vi "Keithley 2002 Scan Read.vi"(1 "delay between\nbus triggers (mS)":dbl=300.0 min=0.0 step=1.0, 2 "scan operation (int:0)":u16(ring) items=["internal", "ratio", "delta"], 4 "count value":dbl=100.0 min=2.0 max=30092.0 step=1.0, 5 "delay (secs)":dbl min=0.0 max=999999.999 format="%.3f", 6 "error in":T2, 7 "timer value (secs)":dbl=0.001 min=0.001 max=999999.999 format="%.3f", 8 "source (imm:1)":u16(ring)=1 items=["hold", "immediate", "timer", "manual", "bus", "trigger link", "external"], 9 "GPIB address":string="16") -> (0 "error out":T2, 3 "measurements":T1(array[cluster]) {"measurement" format="%.6e"})   [LabVIEW 2020]
doc: "This VI is used to configure the Measure Layer (Trigger) and then read the scanning channels. The count value will control the number of measurements taken. The channels (1-10) will be scanned in order. If the count value is more than the number of channels to be scanned, the scan will repeat and read through the channels again.\n\nTo configure the scanning channels, use the Scan Config VI."
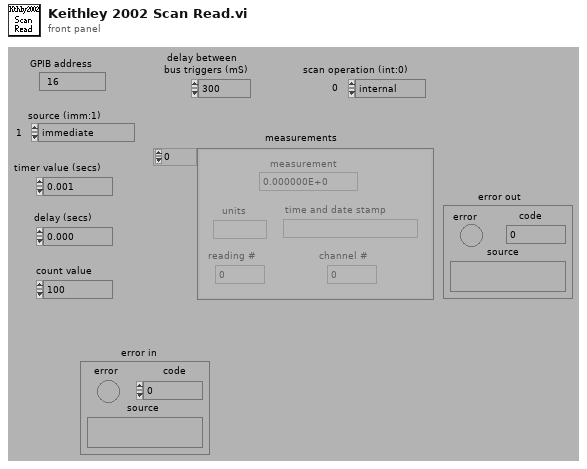
[diagram p1: front panel]
types:
  T1 = cluster{"measurement":dbl, "units":string, "time and date stamp":string, "reading #":dbl, "channel #":dbl}[]
  T2 = cluster{"error":bool, "code":i32, "source":string}
  T3 = cluster{dbl, "read buffer":string, "read buffer":string, dbl, dbl}
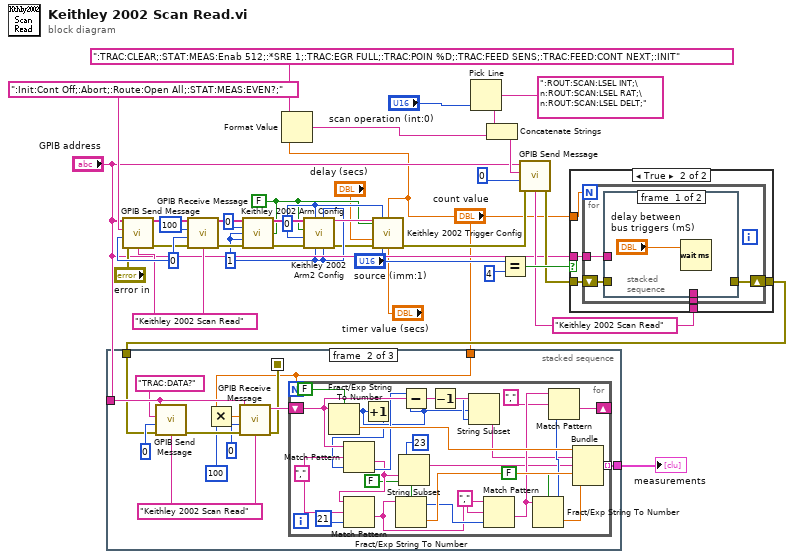
[diagram p0: block diagram]
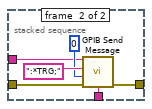
[diagram p3: hidden frame]
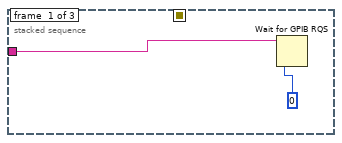
[diagram p4: hidden frame]
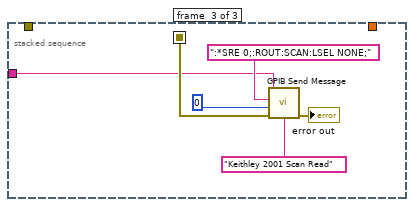
[diagram p5: hidden frame]
diagram:
  w15 = "Keithley 2002 Scan Read"
  w29 = 0
  w8 = 0
  w7 = FALSE
  w10 = 1
  w20 = "Keithley 2002 Scan Read"
  n1 = call "GPIB Send Message.vi"("address string"="GPIB address", "write buffer"=":Init:Cont Off;:Abort;:Route:Open All;:STAT:MEAS:EVEN?;", "source"=w15, "write mode (set END:0)"=w29, "error in"="error in") -> ("error out"=w16:T2)  [unwired: 2 in, 2 out]
  n2 = call "GPIB Receive Message.vi"("address string"="GPIB address", "byte count"=100, "source"=w15, "read mode"=w29, "error in"=w16) -> ("error out"=w14:T2)  [unwired: 2 in, 2 out]
  n3 = call "Keithley 2002 Arm Config.vi"("GPIB address"="GPIB address", "count (set:0)"=0, "count value"=w10, "direction"=w7, "source (imm:1)"=w10, "error in"=w14) -> ("error out"=w11:T2)  [unwired: 9 in]
  n4 = Format Value(format string=":TRAC:CLEAR;:STAT:MEAS:Enab 512;:*SRE 1;:TRAC:EGR FULL;:TRAC:POIN %D;:TRAC:FEED SENS;:TRAC:FEED:CONT NEXT;:INIT", value (0)="count value") -> (output string=w17:string)  [unwired: 1 in]
  n5 = call "Keithley 2002 Arm2 Config.vi"("timer value (secs)"=w10, "count value"=w10, "source (imm:1)"=w10, "count (set:0)"=w8, "error in"=w11, "delay (secs)"=w8, "direction"=w7, "GPIB address"="GPIB address") -> ("error out"=w9:T2)  [unwired: 3 in]
  n6 = call "Keithley 2002 Trigger Config.vi"("GPIB address"="GPIB address", "count (set:0)"=w8, "count value"="count value", "direction"=w7, "delay (secs)"="delay (secs)", "error in"=w9, "source (imm:1)"="source (imm:1)", "timer value (secs)"="timer value (secs)") -> ("error out"=w3:T2)  [unwired: 7 in]
  n7 = Pick Line(multi-line string=":ROUT:SCAN:LSEL INT;\n:ROUT:SCAN:LSEL RAT;\n:ROUT:SCAN:LSEL DELT;", line index="scan operation (int:0)") -> (output string=w25:string)  [unwired: 1 in]
  n8 = Concatenate Strings(w25, w17) -> (w24:string)
  n9 = Equal?(x="source (imm:1)", y=4) -> (x = y?=w23:bool)
  n10 = call "GPIB Send Message.vi"("address string"="GPIB address", "write buffer"=w24, "source"=w20, "write mode (set END:0)"=0, "error in"=w3) -> ("error out"=w19:T2)  [unwired: 2 in, 2 out]
  n11 = case shown="True" w23 {
    tunnel: "count value" -> [_ w38]
    tunnel: [w33 w37] -> w21
    tunnel: w20 -> [_ w36]
    tunnel: "GPIB address" -> [_ w35]
    tunnel: w19 -> [w33 w34]
    frame False {
    }
    frame True {
      n12 = for {
        N: w38 -> [_]
        shift-right: [w40] -> w37
        shift-left: w34 -> [w41]
        tunnel: w36 -> [w39]
        tunnel: w35 -> [w42]
        n13 = stacked-sequence {
          tunnel: w42 -> [_ w47]
          tunnel: w41 -> [_ w46]
          tunnel: [_ w45] -> w40
          tunnel: w39 -> [_ w44]
          frame #0 {
            n14 = Wait (ms)(milliseconds to wait="delay between\nbus triggers (mS)") -> ()  [unwired: 1 out]
          }
          frame #1 {
            n15 = call "GPIB Send Message.vi"("address string"=w47, "write buffer"=":*TRG;", "source"=w44, "write mode (set END:0)"=0, "error in"=w46) -> ("error out"=w45:T2)  [unwired: 2 in, 2 out]
          }
        }
      }
    }
  }
  n16 = stacked-sequence {
    seq-local: [_ w63 _] -> [_ _ w94]
    tunnel: "count value" -> [_ w55 _]
    tunnel: "GPIB address" -> [w50 w61 w93]
    tunnel: w21 -> [_ w53 _]
    tunnel: [_ w52 _] -> w1
    frame #0 {
      n17 = Wait for GPIB RQS(3:0, 4:w50) -> ()  [unwired: 1 in, 2 out]
    }
    frame #1 {
      w60 = "Keithley 2002 Scan Read"
      n18 = call "GPIB Send Message.vi"("address string"=w61, "write buffer"="TRAC:DATA?", "source"=w60, "write mode (set END:0)"=0, "error in"=w53) -> ("error out"=w62:T2)  [unwired: 2 in, 2 out]
      n19 = Multiply(x=w55, y=100) -> (x*y=w54:dbl)
      n20 = call "GPIB Receive Message.vi"("address string"=w61, "byte count"=w54, "source"=w60, "read mode"=0, "error in"=w62) -> ("read buffer"=w64:string, "error out"=w63:T2)  [unwired: 2 in, 1 out]
      n21 = for {
        N: w55 -> [_]
        shift-right: [w80] -> _
        shift-left: w64 -> [w79]
        tunnel: [w68] -> w52 mode=indexing
        w85 = ","
        n22 = Fract/Exp String To Number(use system decimal point (T)=FALSE, string=w79) -> (offset past number=w74:i32, number=w90:dbl)  [unwired: 2 in]
        n23 = Increment(x=w74) -> (x+1=w73:i32)
        n24 = Match Pattern(string=w79, regular expression=w85, offset (0)=w73) -> (after substring=w72:string, offset past match=w77:i32)  [unwired: 2 out]
        n25 = Match Pattern(string=w72, regular expression=w85, offset (0)=21) -> (after substring=w86:string)  [unwired: 3 out]
        n26 = Fract/Exp String To Number(use system decimal point (T)=FALSE, string=w86) -> (offset past number=w87:i32, number=w89:dbl)  [unwired: 2 in]
        n27 = String Subset(string=w72, length (rest)=23) -> (substring=w71:string)  [unwired: 1 in]
        n28 = Subtract(x=w77, y=w74) -> (x-y=w78:i32)
        n29 = Decrement(x=w78) -> (x-1=w75:i32)
        n30 = String Subset(string=w79, offset (0)=w74, length (rest)=w75) -> (substring=w76:string)
        n31 = Match Pattern(string=w86, regular expression=",", offset (0)=w87) -> (after substring=w83:string)  [unwired: 3 out]
        n32 = Fract/Exp String To Number(use system decimal point (T)=FALSE, string=w83) -> (offset past number=w82:i32, number=w88:dbl)  [unwired: 2 in]
        n33 = Match Pattern(string=w83, regular expression=",", offset (0)=w82) -> (after substring=w80:string)  [unwired: 3 out]
        n34 = Bundle(w90, "read buffer"=w76, "read buffer"=w71, w89, w88) -> (w68:T3)  [unwired: 1 in]
      }
    }
    frame #2 {
      n35 = call "GPIB Send Message.vi"("address string"=w93, "write buffer"=":*SRE 0;:ROUT:SCAN:LSEL NONE;", "source"="Keithley 2001 Scan Read", "write mode (set END:0)"=0, "error in"=w94) -> ("error out"=→"error out":T2)  [unwired: 2 in, 2 out]
    }
  }
  "measurements" <- w1
